vi "TW Basic Generate LV Icon Text Layer.vi"(8 "error in (no error)":errorcluster, 9 "Text color":u32(colorbox), 10 "Background":u32(colorbox)=7208704, 11 "Name":string) -> (0 "error out":errorcluster, 2 "Picture":picture, 3 "Icon.lvlclass out":refnum<class "Icon.lvclass">)   [LabVIEW 2021]
doc: "Basic example that shows how to set the Text Layer"
uses:
  <vilib>/LabVIEW Icon API/lv_icon/Classes/Icon/Icon.lvclass
  <vilib>/LabVIEW Icon API/API_Rectangle Dimension.ctl
  <vilib>/LabVIEW Icon API/API_Text.ctl
  <vilib>/LabVIEW Icon API/API_Rectangle Colors.ctl
  <vilib>/LabVIEW Icon API/LabVIEW Icon API.lvlib
  <vilib>/LabVIEW Icon API/lv_icon/Controls/Alignment.ctl
  <vilib>/LabVIEW Icon API/API_Text Colors.ctl
  <vilib>/LabVIEW Icon API/API_Test Settings.ctl
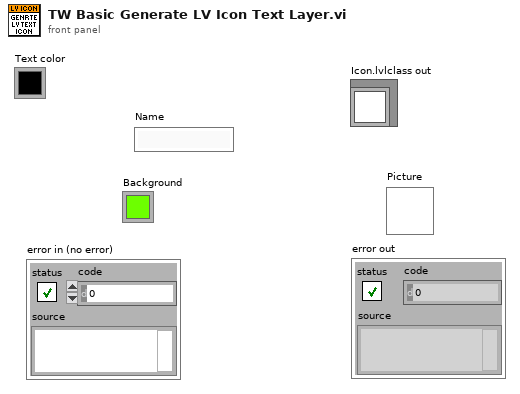
[diagram p1: front panel]
types:
  T1 = typedef "LabVIEW Icon API.lvlib/API_Test Settings.ctl" = cluster{"Font":string, "Alignment":T2, "Size":u8, "Center text":bool, "Capitalize text":bool, "Text color":T3}
  T2 = typedef "Alignment.ctl" = u16
  T3 = typedef "LabVIEW Icon API.lvlib/API_Text Colors.ctl" = cluster{"Line 1 color":u32, "Line 2 color":u32, "Line 3 color":u32, "Line 4 color":u32}
  T4 = typedef "LabVIEW Icon API.lvlib/API_Rectangle Colors.ctl" = cluster{"Border":u32, "Background":u32}
  T5 = typedef "LabVIEW Icon API.lvlib/API_Text.ctl" = cluster{"Line 1 text":string, "Line 2 text":string, "Line 3 text":string, "Line 4 text":string}
  T6 = typedef "LabVIEW Icon API.lvlib/API_Rectangle Dimension.ctl" = cluster{"Width":i16, "Height":i16}
  T7 = typedef "LabVIEW Icon API.lvlib/API_User Layer Data.ctl" = cluster{"Layer name":string, "Origin":T8, "Icon image data":T9}
  T8 = typedef "LVPoint32TypeDef.ctl" = cluster{"Horizontal":i32, "Vertical":i32}
  T9 = typedef "imagedata.ctl" = cluster{"image type":i32, "image depth":i32, "image":u8[], "mask":u8[], "colors":u32[], "Rectangle":cluster{"left":i16, "top":i16, "right":i16, "bottom":i16}}
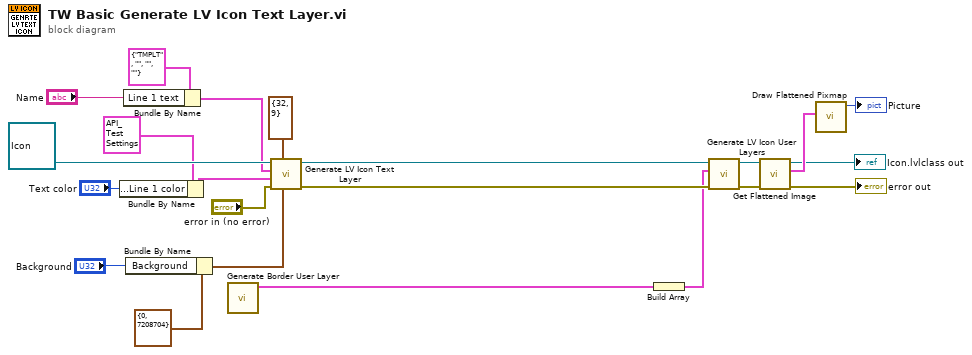
[diagram p0: block diagram]
diagram:
  n1 = Bundle By Name(cluster=T1 {"Font"="Small Fonts", "Alignment"=1, "Size"=8, "Center text"=TRUE, "Capitalize text"=TRUE, "Text color"={"Line 1 color"=0, "Line 2 color"=0, "Line 3 color"=0, "Line 4 color"=0}} ("Text settings"), "Text color.Line 1 color"="Text color") -> (w2:T1)
  n2 = Bundle By Name(cluster=T5 {"Line 1 text"="TMPLT", "Line 2 text"="", "Line 3 text"="", "Line 4 text"=""} ("Text"), "Line 1 text"="Name") -> (w7:T5)
  n3 = Bundle By Name(cluster=T4 {"Border"=0, "Background"=7208704} ("Rectangle colors (black, white)"), "Background"="Background") -> (w4:T4)
  n4 = call <vilib>:"Generate Border User Layer.vi"() -> ("User Layer data"=w13:T7)  [unwired: 11 in]
  n5 = call <vilib>:"Generate LV Icon Text Layer.vi"("Rectangle colors (black, white)"=w4, "Rectangle dimension (32,32)"=T6 {"Width"=32, "Height"=9}, "error in (no error)"="error in (no error)", "Text settings"=w2, "Text"=w7, "Icon in"=refnum<class "Icon.lvclass"> refnum ("Icon.lvclass in")) -> ("error out"=w19:errorcluster, "Icon out"=w18:refnum<class "Icon.lvclass">)  [unwired: 4 in]
  n6 = Build Array(w13) -> (w12:T7[])
  n7 = call <vilib>:"Generate LV Icon User Layers.vi"("error in (no error)"=w19, "User layers"=w12, "Icon in"=w18) -> ("error out"=w16:errorcluster, "Icon out"=w14:refnum<class "Icon.lvclass">)  [unwired: 7 in]
  n8 = call <vilib>:"Get Flattened Image.vi"("error in (no error)"=w16, "lv_icon.lvlib:Icon.lvclass in"=w14) -> ("error out"=→"error out":errorcluster, "Color Image"=w20:T9, "lv_icon.lvlib:Icon.lvclass out"=→"Icon.lvlclass out":refnum<class "Icon.lvclass">)  [unwired: 6 in, 1 out]
  n9 = call <vilib>:"Draw Flattened Pixmap.vi"("image data"=w20) -> ("new picture"=→"Picture":picture)  [unwired: 8 in]
